vi "makeDirectory.vi"(8 "error in":errorcluster caption="에러 입력", 10 "설정 디렉토리":string[](array[string]), 11 "파일저장경로":path) -> (0 "error out":errorcluster caption="에러 출력")   [LabVIEW 2018]
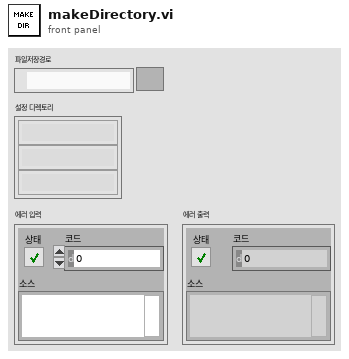
[diagram p1: front panel]
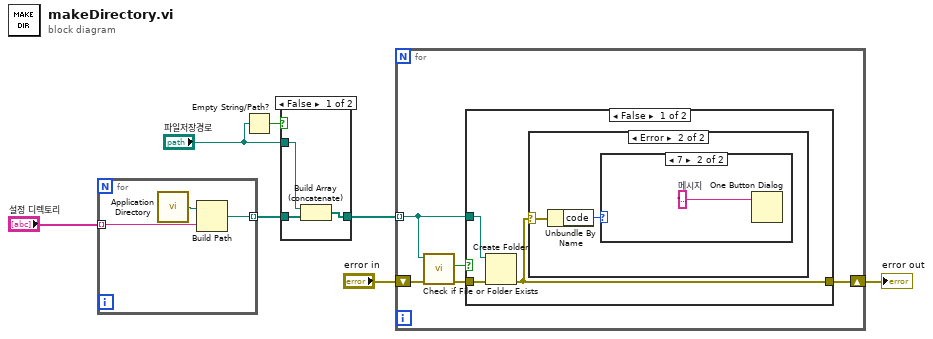
[diagram p0: block diagram]
diagram:
  n1 = for {
    tunnel: "설정 디렉토리" -> [w9] mode=indexing
    tunnel: [w8] -> w7 mode=indexing
    n2 = call <vilib>:"Application Directory.vi"() -> ("Application Directory"=w10:path)
    n3 = Build Path(base path=w10, name or relative path=w9) -> (appended path=w8:path)
  }
  n4 = Empty String/Path?(string/path="파일저장경로") -> (empty?=w3:bool)
  n5 = case shown="False" w3 {
    tunnel: w7 -> [w13 w14]
    tunnel: [w12 w14] -> w5
    tunnel: "파일저장경로" -> [w11 _]
    frame False {
      n6 = Build Array (concatenate)(w11, w13) -> (w12:path[])
    }
    frame True {
    }
  }
  n7 = for {
    tunnel: w5 -> [w18] mode=indexing
    shift-right: [w16] -> w1
    shift-left: "error in" -> [w17]
    n8 = call <vilib>:"Check if File or Folder Exists.vi"("error in (no error)"=w17, "path"=w18) -> ("error out"=w15:errorcluster, "file or folder exists?"=w19:bool)  [unwired: 7 in, 1 out]
    n9 = case shown="False" w19 {
      tunnel: w18 -> [w22 _]
      tunnel: [w21 w26] -> w16
      tunnel: w15 -> [w20 w26]
      frame False {
        n10 = Create Folder(path (use dialog)=w22, error in=w20) -> (error out=w21:errorcluster)  [unwired: 1 in, 2 out]
        n11 = case shown="Error" w21 {
          selector: w21 -> [_ w24]
          frame No Error {
          }
          frame Error {
            n12 = Unbundle By Name(w24) -> ("code"=w23:i32)
            n13 = case shown="7" w23 {
              frame Default {
              }
              frame 7 {
                w25 = "디렉토리 생성 에러 "  # 메시지
                n14 = One Button Dialog(message=w25) -> ()  [unwired: 1 in, 1 out]
              }
            }
          }
        }
      }
      frame True {
      }
    }
  }
  "error out" <- w1
